vi "Autonomous Independent.vi"   [LabVIEW 2013]
doc: "This VI is called when autonomous begins, and will automatically be terminated when autonomous ends. You can carry out timed or sensor driven robot movement independently without needing to return to the caller."
uses:
  <vilib>/Rock Robotics/WPI/Solenoid/WPI_SolenoidValue.ctl
  Robot Global Data.vi
  <vilib>/Rock Robotics/WPI/RobotDrive/WPI_RobotDriveGetSetRefNum.vi
  <vilib>/Rock Robotics/WPI/Solenoid/WPI_SolenoidSetEnum.vi
  <vilib>/Rock Robotics/WPI/RobotDrive/WPI_RobotDriveArcadeDrive_Standard(NoSaturation).vi
  <vilib>/Rock Robotics/WPI/Solenoid/Deprecated/WPI_SolenoidGetBool.vi
  <vilib>/Rock Robotics/WPI/Joystick/WPI_JoystickGetSetRefNum.vi
panel:
  # "Be sure to right-click and choose Data Operations>>Make Current Value default if you want to save the array values with the VI"
types:
  T1 = typedef "WPI_JoystickDevRef.ctl" = cluster{"Device":T2}
  T2 = typedef "WPI_JoystickDeviceEnum.ctl" = enum16{"USB 1", "USB 2", "USB 3", "USB 4", "Kinect 1", "Kinect 2"}
  T3 = cluster{"axis 1 (x)":dbl, "axis 2 (y)":dbl, "axis 3 (throttle)":dbl, "axis 4":dbl, "axis 5":dbl, "axis 6":dbl}
  T4 = typedef "WPI_MotorControlDeviceRef.ctl" = cluster{"DeviceStatus":errorcluster, "Type":enum16{"PWM", "CAN"}, "PWM":cluster{"Digital Module":T5, "PWM Channel":T6, "DeadBand":T7}, "CAN":cluster{"Device Number":u8, "Control Mode":T8, "Semaphore":T9, "Max Vout":dbl}, "Invert":bool, "TransformRef":T10, "InvTransformRef":T10}
  T5 = typedef "FPGA_TypedefDigitalModule.ctl" = enum16{"Digital Module 1", "Digital Module 2"}
  T6 = typedef "FPGA_DIOPWMChannel.ctl" = enum8{"PWM 1", "PWM 2", "PWM 3", "PWM 4", "PWM 5", "PWM 6", "PWM 7", "PWM 8", "PWM 9", "PWM 10", "Invalid"}
  T7 = typedef "WPI_PWMDeadband.ctl" = cluster{"Name":string, "maxPositivePwm":i32, "minPositivePwm":i32, "centerPwm":i32, "maxNegativePwm":i32, "minNegativePwm":i32, "angularRange":u16}
  T8 = typedef "WPI_CANJaguar_ControlMode.ctl" = enum8{"Percent VBus", "Current", "Speed", "Position", "Voltage"}
  T9 = typedef "Semaphore RefNum" = refnum<k1>
  T10 = typedef "WPI_PWMTransform_ConPane.ctl" = refnum<vi>
  T11 = typedef "WPI_SolenoidDevRef.ctl" = cluster{"DevStatus":errorcluster, "Solenoid Module":T12, "Forward Solenoid Channel":T13, "Reverse Solenoid Channel":T13}
  T12 = typedef "FPGA_TypedefSolenoidModule.ctl" = enum16{"Solenoid Module 1", "Solenoid Module 2"}
  T13 = typedef "WPI_SolenoidChannel.ctl" = enum8{"Solenoid 1", "Solenoid 2", "Solenoid 3", "Solenoid 4", "Solenoid 5", "Solenoid 6", "Solenoid 7", "Solenoid 8", "Invalid"}
  T14 = typedef "WPI_RobotDriveDevRef.ctl" = cluster{"DevStatus":errorcluster, "Motors[]":T4[], "Square Inputs":bool, "Max Output":dbl, "Isochronous":bool}
  T15 = typedef "WPI_SolenoidValue.ctl" = enum16{"Off", "On", "Forward", "Reverse"}
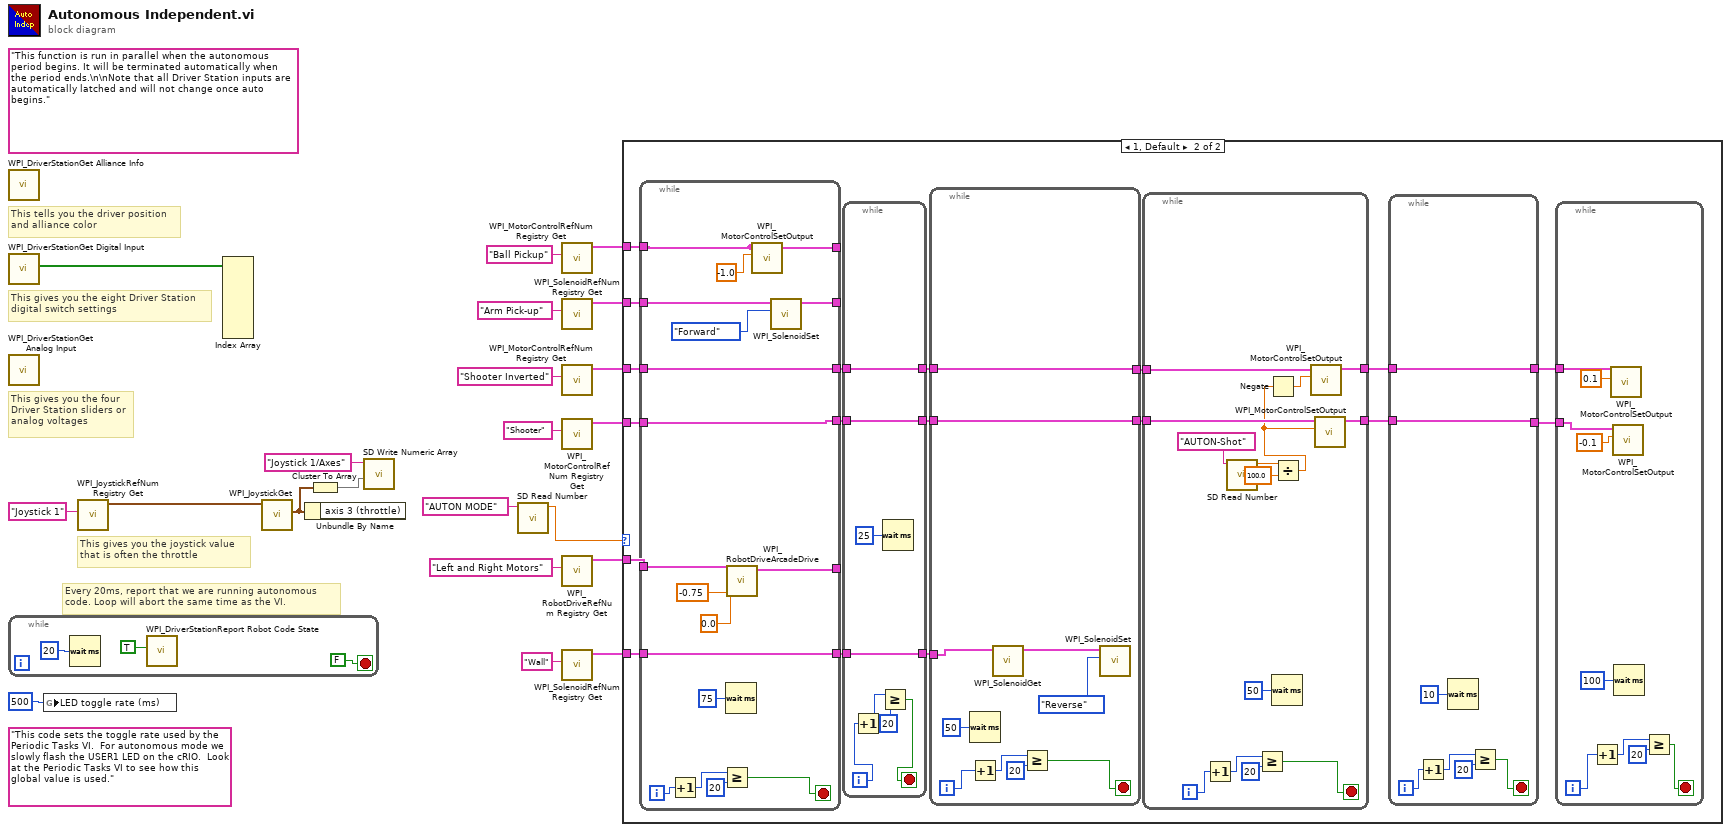
[diagram p0: block diagram]
diagram:
  (unwired) "This code sets the toggle rate used by the Periodic Tasks VI.  For autonomous mode we slowly flash the USER1 LED on the cRIO.  Look at the Periodic Tasks VI to see how this global value is used."
  (unwired) "This function is run in parallel when the autonomous period begins. It will be terminated automatically when the period ends.\n\nNote that all Driver Station inputs are automatically latched and will not change once auto begins."
  # "Every 20ms, report that we are running autonomous\ncode. Loop will abort the same time as the VI."
  # "This gives you the joystick value\nthat is often the throttle"
  # "This tells you the driver position\nand alliance color"
  # "This gives you the eight Driver Station\ndigital switch settings"
  # "This gives you the four\nDriver Station sliders or\nanalog voltages"
  n1 = call <vilib>:"WPI_DriverStationGet Alliance Info.vi"() -> ()  [unwired: 12 out]
  n2 = call <vilib>:"WPI_DriverStationGet Digital Input.vi"() -> ("Driver Station Digital Input (1-8)"=w21:bool[])  [unwired: 11 out]
  n3 = call <vilib>:"WPI_DriverStationGet Analog Input.vi"() -> ()  [unwired: 12 out]
  n4 = while {
    stop <- FALSE stop-if-true
    n5 = Wait (ms)(milliseconds to wait=u32 20) -> ()  [unwired: 1 out]
    n6 = call <vilib>:"WPI_DriverStationReport Robot Code State.vi"("Autonomous"=TRUE) -> ()  [unwired: 10 in, 1 out]
  }
  n7 = global write "Robot Global Data.vi" "LED toggle rate (ms)"(u32 500 ("LED ms toggle rate")) -> ()
  n8 = call <vilib>:"WPI_JoystickRefNum Registry Get.vi"("refnum name"="Joystick 1") -> ("JoystickDevRef"=w19:T1)  [unwired: 1 in, 9 out]
  n9 = Index Array(array=w21) -> ()  [unwired: 8 in, 8 out]
  n10 = call <vilib>:"WPI_JoystickGet.vi"("JoystickDevRef"=w19) -> ("Axes"=w16:T3)  [unwired: 1 in, 5 out]
  n11 = Unbundle By Name(w16) -> ()  [unwired: 1 out]
  n12 = Cluster To Array(cluster=w16) -> (array=w17:dbl[])
  n13 = call <vilib>:"SD Write Numeric Array.vi"("Numeric Array"=w17, "Name"="Joystick 1/Axes") -> ()  [unwired: 8 in, 2 out]
  n14 = call <vilib>:"SD Read Number.vi"("Name"="AUTON MODE") -> ("Numeric"=w13:dbl)  [unwired: 8 in, 2 out]
  n15 = call <vilib>:"WPI_MotorControlRefNum Registry Get.vi"("refnum name"="Ball Pickup") -> ("MotorControlDevRef"=w1:T4)  [unwired: 9 in, 1 out]
  n16 = call <vilib>:"WPI_SolenoidRefNum Registry Get.vi"("refnum name"="Arm Pick-up") -> ("SolenoidDevRef"=w2:T11)  [unwired: 9 in, 1 out]
  n17 = call <vilib>:"WPI_MotorControlRefNum Registry Get.vi"("refnum name"="Shooter Inverted") -> ("MotorControlDevRef"=w3:T4)  [unwired: 9 in, 1 out]
  n18 = call <vilib>:"WPI_MotorControlRefNum Registry Get.vi"("refnum name"="Shooter") -> ("MotorControlDevRef"=w4:T4)  [unwired: 9 in, 1 out]
  n19 = call <vilib>:"WPI_RobotDriveRefNum Registry Get.vi"("refnum name"="Left and Right Motors") -> ("RobotDriveDevRef"=w6:T14)  [unwired: 9 in, 1 out]
  n20 = call <vilib>:"WPI_SolenoidRefNum Registry Get.vi"("refnum name"="Wall") -> ("SolenoidDevRef"=w5:T11)  [unwired: 9 in, 1 out]
  n21 = case shown="1, Default" w13 {
    tunnel: w6 -> [_ w42]
    tunnel: w5 -> [_ w31]
    tunnel: w4 -> [_ w41]
    tunnel: w3 -> [_ w40]
    tunnel: w2 -> [_ w39]
    tunnel: w1 -> [_ w38]
    frame 0 {
    }
    frame 1, Default {
      n22 = while {
        tunnel: w42 -> [w102]
        tunnel: [w100] -> _
        tunnel: [w99] -> w28
        tunnel: w41 -> [w99]
        tunnel: w40 -> [w98]
        tunnel: [w98] -> w25
        tunnel: w39 -> [w93]
        tunnel: w38 -> [w92]
        tunnel: [w92] -> _
        tunnel: [w93] -> _
        tunnel: [w95] -> w30
        tunnel: w31 -> [w95]
        i -> [w106]
        stop <- w103 stop-if-true
        n23 = Increment(x=w106) -> (x+1=w105:i32)
        n24 = Greater Or Equal?(x=w105, y=20) -> (x >= y?=w103:bool)
        n25 = Wait (ms)(milliseconds to wait=u32 75) -> ()  [unwired: 1 out]
        n26 = call-poly <vilib>:"WPI_RobotDriveArcadeDrive.vi"("Y axis value"=-0.75, "X axis value"=0.0, "RobotDriveDevRef"=w102) -> ("RobotDriveDevRef"=w100:T14)  [unwired: 6 in, 2 out]
        n27 = call <vilib>:"WPI_MotorControlSetOutput.vi"("Output"=-1.0, "MotorControlDevRef"=w92) -> ()  [unwired: 7 in, 3 out]
        n28 = call-poly <vilib>:"WPI_SolenoidSet.vi"("Value"=WPI_SolenoidValue."Forward", "SolenoidDevRef"=w93) -> ()  [unwired: 8 in, 2 out]
      }
      n29 = while {
        tunnel: w30 -> [w50]
        tunnel: [w50] -> w29
        tunnel: w28 -> [w49]
        tunnel: [w49] -> w27
        tunnel: [w48] -> w26
        tunnel: w25 -> [w48]
        i -> [w45]
        stop <- w44 stop-if-true
        n30 = Increment(x=w45) -> (x+1=w46:i32)
        n31 = Greater Or Equal?(x=w46, y=20) -> (x >= y?=w44:bool)
        n32 = Wait (ms)(milliseconds to wait=u32 25) -> ()  [unwired: 1 out]
      }
      n33 = while {
        tunnel: w27 -> [w85]
        tunnel: w26 -> [w86]
        tunnel: [w86] -> w37
        tunnel: [w85] -> w36
        tunnel: w29 -> [w83]
        i -> [w88]
        stop <- w87 stop-if-true
        n34 = Wait (ms)(milliseconds to wait=u32 50) -> ()  [unwired: 1 out]
        n35 = Increment(x=w88) -> (x+1=w89:i32)
        n36 = call-poly <vilib>:"WPI_SolenoidGet.vi"("SolenoidDevRef"=w83) -> ("SolenoidDevRef"=w81:T11)  [unwired: 8 in, 2 out]
        n37 = Greater Or Equal?(x=w89, y=20) -> (x >= y?=w87:bool)
        n38 = call-poly <vilib>:"WPI_SolenoidSet.vi"("Value"=WPI_SolenoidValue."Reverse", "SolenoidDevRef"=w81) -> ()  [unwired: 8 in, 2 out]
      }
      n39 = while {
        tunnel: w37 -> [w76]
        tunnel: w36 -> [w75]
        tunnel: [w74] -> w35
        tunnel: [w73] -> w34
        i -> [w78]
        stop <- w77 stop-if-true
        n40 = Increment(x=w78) -> (x+1=w80:i32)
        n41 = call <vilib>:"SD Read Number.vi"("Name"="AUTON-Shot") -> ("Numeric"=w69:dbl)  [unwired: 8 in, 2 out]
        n42 = Greater Or Equal?(x=w80, y=20) -> (x >= y?=w77:bool)
        n43 = Wait (ms)(milliseconds to wait=u32 50) -> ()  [unwired: 1 out]
        n44 = Divide(x=w69, y=100.0) -> (x/y=w68:dbl)
        n45 = Negate(x=w68) -> (-x=w70:dbl)
        n46 = call <vilib>:"WPI_MotorControlSetOutput.vi"("Output"=w70, "MotorControlDevRef"=w76) -> ("MotorControlDevRef"=w73:T4)  [unwired: 7 in, 2 out]
        n47 = call <vilib>:"WPI_MotorControlSetOutput.vi"("Output"=w68, "MotorControlDevRef"=w75) -> ("MotorControlDevRef"=w74:T4)  [unwired: 7 in, 2 out]
      }
      n48 = while {
        tunnel: w35 -> [w62]
        tunnel: w34 -> [w61]
        tunnel: [w62] -> w32
        tunnel: [w61] -> w33
        i -> [w63]
        stop <- w64 stop-if-true
        n49 = Increment(x=w63) -> (x+1=w65:i32)
        n50 = Wait (ms)(milliseconds to wait=u32 10) -> ()  [unwired: 1 out]
        n51 = Greater Or Equal?(x=w65, y=20) -> (x >= y?=w64:bool)
      }
      n52 = while {
        tunnel: w33 -> [w58]
        tunnel: w32 -> [w59]
        i -> [w53]
        stop <- w52 stop-if-true
        n53 = Increment(x=w53) -> (x+1=w55:i32)
        n54 = call <vilib>:"WPI_MotorControlSetOutput.vi"("Output"=0.1, "MotorControlDevRef"=w58) -> ()  [unwired: 7 in, 3 out]
        n55 = call <vilib>:"WPI_MotorControlSetOutput.vi"("Output"=-0.1, "MotorControlDevRef"=w59) -> ()  [unwired: 7 in, 3 out]
        n56 = Wait (ms)(milliseconds to wait=u32 100) -> ()  [unwired: 1 out]
        n57 = Greater Or Equal?(x=w55, y=20) -> (x >= y?=w52:bool)
      }
    }
  }
